vi "Get Log Column Headers.vi"() -> (2 "Headers String":string)   [LabVIEW 2015]
uses:
  Sensors/Sensor Enum.ctl
  Sensors/Sensor Data Global Action.ctl
panel:
  in  "Sensor Name":T1
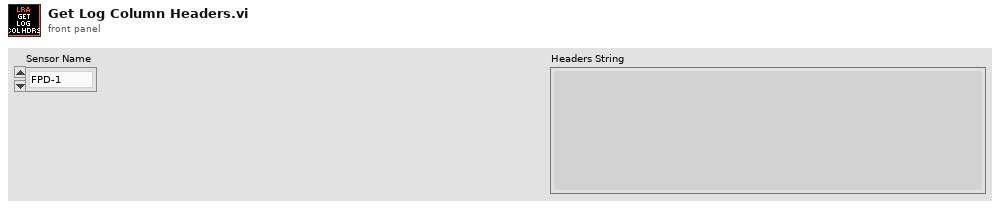
[diagram p1: front panel]
types:
  T1 = typedef "Sensor Enum.ctl" = enum16{"FPD-1", "FPD-2", "FPD-3", "OPD-1", "OPD-2", "OPD-3", "AP-1", "PC-1", "PC-2", "VBAT", "VCOMP", "ICOMP", "TC-1", "TC-COMP"}
  T2 = typedef "Sensor Data Global Action.ctl" = enum16{"Get Data", "Decode & Store Data"}
  T3 = typedef "Transducer Calibration Display.ctl" = cluster{"Value":dbl, "Raw":dbl, "Scaled":dbl, "Sensor Name":T1, "Port":u32}
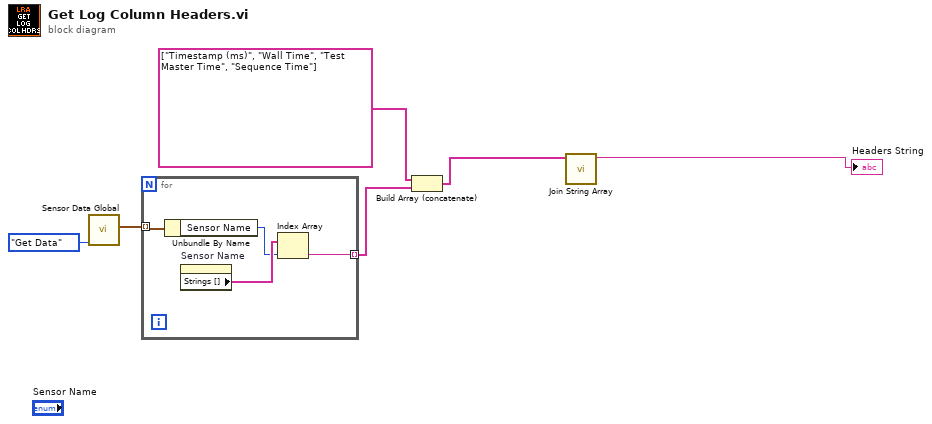
[diagram p0: block diagram]
diagram:
  n1 = call "Sensor Data Global.vi"("Command"=Sensor_Data_Global_Action."Get Data") -> ("Sensor Data"=w5:T3[])  [unwired: 10 in]
  n2 = for {
    tunnel: w5 -> [w10] mode=indexing
    tunnel: [w7] -> w3 mode=indexing
    n3 = Unbundle By Name(w10) -> ("Sensor Name"=w8:T1)
    n4 = property on="Sensor Name" class="Enum (strict)"() -> ("Strings []"=w9:string[])  [unwired: 2 in, 2 out]
    n5 = Index Array(array=w9, index=w8) -> (element=w7:string)
  }
  n6 = Build Array (concatenate)(string[] ["Timestamp (ms)", "Wall Time", "Test Master Time", "Sequence Time"], w3) -> (w2:string[])
  n7 = call "Join String Array.vi"("Array"=w2) -> ("String"=→"Headers String":string)  [unwired: 10 in]
